vi "Get Status.vi"(8 "error in (no error)":errorcluster) -> (0 "error out":errorcluster, 3 "Status":T1)   [LabVIEW 2020, in "Manipulator CLI Driver.lvlib"]
uses:
  Manipulator Status.ctl
  Manipulator CLI Driver.lvlib
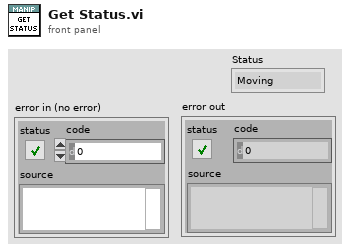
[diagram p1: front panel]
types:
  T1 = typedef "Manipulator CLI Driver.lvlib/Manipulator Status.ctl" = enum16{"Moving", "Done", "Aborted", "Error", "No Status"}
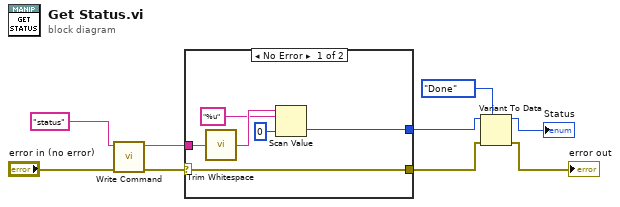
[diagram p0: block diagram]
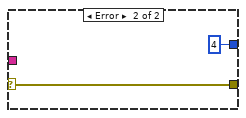
[diagram p2: hidden frame]
diagram:
  n1 = call "Write Command.vi"("error in (no error)"="error in (no error)", "command"="status") -> ("error out"=w7:errorcluster, "standard output"=w6:string)  [unwired: 7 in, 1 out]
  n2 = case shown="No Error" w7 {
    selector: w7 -> [w15 w17]
    tunnel: [w15 w17] -> w4
    tunnel: w6 -> [w14 _]
    tunnel: [w11 4 ("default (0 dbl)")] -> w1
    frame No Error {
      n3 = call <vilib>:"Trim Whitespace.vi"("string"=w14) -> ("trimmed string"=w13:string)  [unwired: 1 in]
      n4 = Scan Value(string=w13, format string="%u", default (0 dbl)=0) -> (value=w11:i32)  [unwired: 1 out]
    }
    frame Error {
    }
  }
  n5 = Variant To Data(error in=w4, type=Manipulator_Status."Done", Variant=w1) -> (data=→"Status":T1, error out=→"error out":errorcluster)
